vi "Create Data Row.vi"(0 "TestRunning?":bool, 1 "Steps":i32, 2 "StepIndex":i32, 3 "SkipStep":bool, 5 "DataCluster":T2, 7 "table.Data":string[][](array[string]), 9 "CommandCluster":T1, 11 "Controller?":bool, 12 "Serial Number":string) -> (4 "DataRow":string[](array[string]), 15 "LastDataTime":i64)   [LabVIEW 2013]
uses:
  TypeDef/DataCluster.ctl
  TypeDef/Command Cluster.ctl
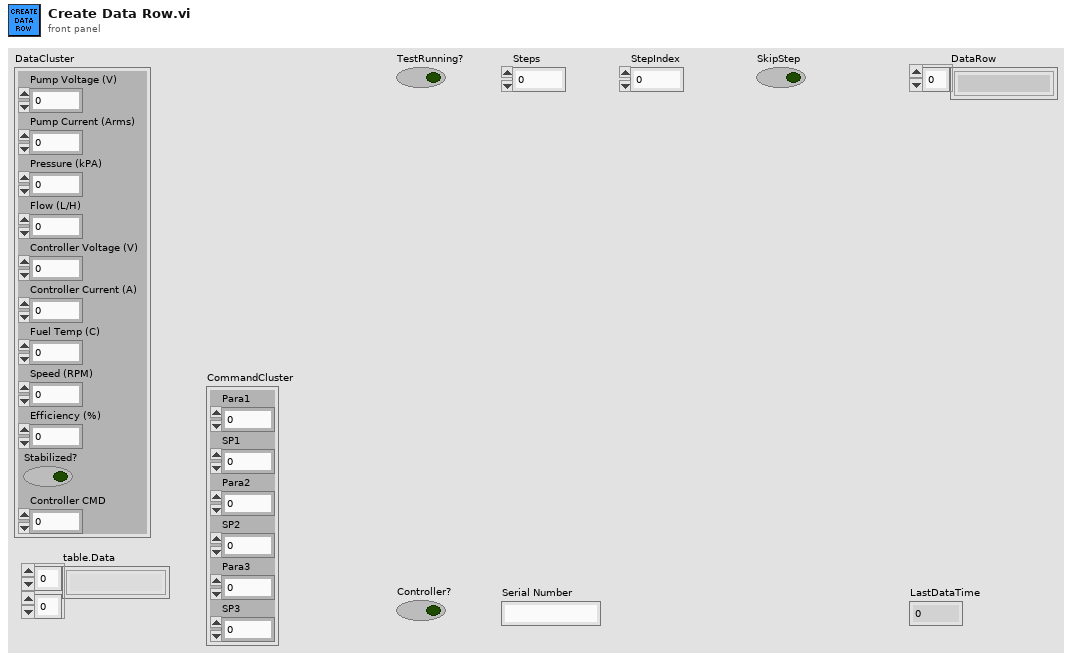
[diagram p1: front panel]
types:
  T1 = typedef "Command Cluster.ctl" = cluster{"Para1":i32, "SP1":dbl, "Para2":i32, "SP2":dbl, "Para3":i32, "SP3":dbl}
  T2 = typedef "DataCluster.ctl" = cluster{"Pump Voltage (V)":dbl, "Pump Current (Arms)":dbl, "Pressure (kPA)":dbl, "Flow (L/H)":dbl, "Controller Voltage (V)":dbl, "Controller Current (A)":dbl, "Fuel Temp (C)":dbl, "Speed (RPM)":dbl, "Efficiency (%)":dbl, "Stabilized?":bool, "Controller CMD":dbl}
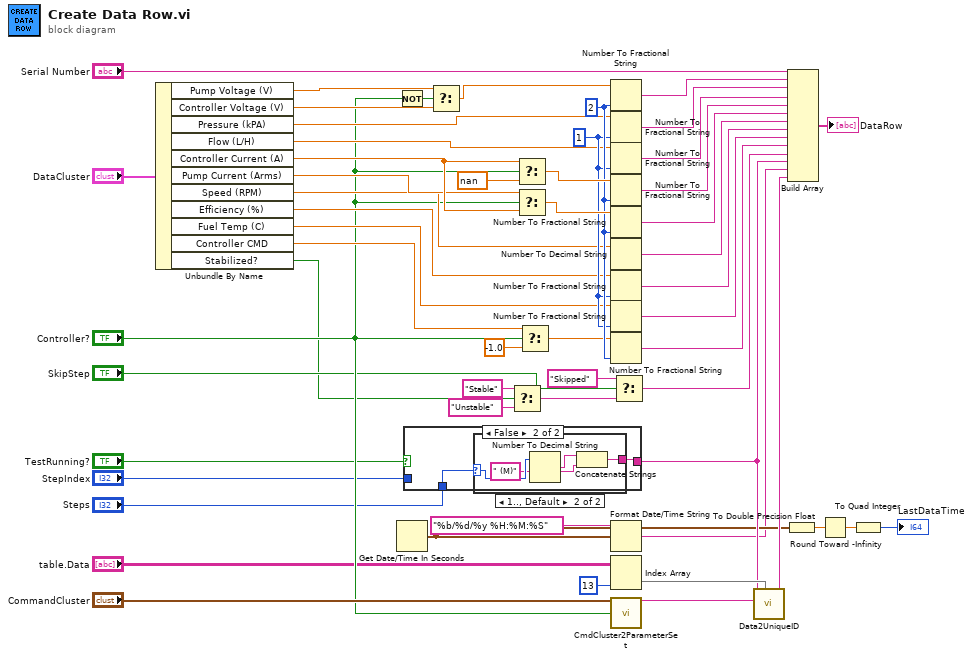
[diagram p0: block diagram]
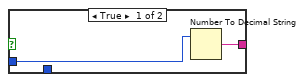
[diagram p2: hidden frame]
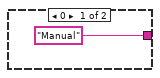
[diagram p3: hidden frame]
diagram:
  w35 = i16 1 ("precision (6)")
  w37 = i16 2 ("precision (6)")
  n1 = Unbundle By Name("DataCluster") -> ("Pump Voltage (V)"=w20:dbl, "Controller Voltage (V)"=w19:dbl, "Pressure (kPA)"=w18:dbl, "Flow (L/H)"=w17:dbl, "Controller Current (A)"=w16:dbl, "Pump Current (Arms)"=w15:dbl, "Speed (RPM)"=w14:dbl, "Efficiency (%)"=w13:dbl, "Fuel Temp (C)"=w12:dbl, "Controller CMD"=w11:dbl, "Stabilized?"=w1:bool)
  n2 = Not(x="Controller?") -> (.not. x?=w54:bool)
  n3 = Get Date/Time In Seconds() -> (seconds since 1Jan1904=w46:timestamp)
  n4 = case shown="False" "TestRunning?" {
    tunnel: "StepIndex" -> [w56 _]
    tunnel: [w57 w59] -> w52
    tunnel: "Steps" -> [_ w58]
    frame True {
      n5 = Number To Decimal String(number=w56) -> (decimal integer string=w57:string)  [unwired: 1 in]
    }
    frame False {
      n6 = case shown="1.., Default" w58 {
        selector: w58 -> [_ w62]
        tunnel: ["Manual" w63] -> w59
        frame 0 {
        }
        frame 1.., Default {
          n7 = Number To Decimal String(number=w62) -> (decimal integer string=w64:string)  [unwired: 1 in]
          n8 = Concatenate Strings(w64, " (M)") -> (w63:string)
        }
      }
    }
  }
  n9 = Select(t=w20, s=w54, f=w19) -> (s? t:f=w29:dbl)
  n10 = Select(t="Stable", s=w1, f="Unstable") -> (s? t:f=w31:string)
  n11 = Select(t=w16, s="Controller?", f=nan) -> (s? t:f=w48:dbl)
  n12 = Select(t=w15, s="Controller?", f=w16) -> (s? t:f=w49:dbl)
  n13 = Select(t=w11, s="Controller?", f=-1.0) -> (s? t:f=w28:dbl)
  n14 = Number To Fractional String(number=w29, precision (6)=w37) -> (F-format string=w23:string)  [unwired: 2 in]
  n15 = Number To Fractional String(number=w18, precision (6)=w35) -> (F-format string=w33:string)  [unwired: 2 in]
  n16 = Number To Fractional String(number=w17, precision (6)=w35) -> (F-format string=w34:string)  [unwired: 2 in]
  n17 = Number To Fractional String(number=w48, precision (6)=w37) -> (F-format string=w24:string)  [unwired: 2 in]
  n18 = Number To Fractional String(number=w49, precision (6)=w37) -> (F-format string=w38:string)  [unwired: 2 in]
  n19 = Number To Decimal String(number=w14) -> (decimal integer string=w36:string)  [unwired: 1 in]
  n20 = Number To Fractional String(number=w13, precision (6)=w35) -> (F-format string=w39:string)  [unwired: 2 in]
  n21 = Number To Fractional String(number=w12, precision (6)=w35) -> (F-format string=w40:string)  [unwired: 2 in]
  n22 = Number To Fractional String(number=w28, precision (6)=w37) -> (F-format string=w41:string)  [unwired: 2 in]
  n23 = Format Date/Time String(time format string (%c)="%b/%d/%y %H:%M:%S", seconds (now)=w46) -> (date/time string=w42:string)  [unwired: 1 in]
  n24 = Index Array(array="table.Data", index (col)=13 ("disabled index (col)")) -> (element=w55:string[])  [unwired: 1 in]
  n25 = call "CmdCluster2ParameterSet.vi"("CMDCluster"="CommandCluster", "Controller?"="Controller?") -> ("ParameterSet"=w51:string)  [unwired: 13 in]
  n26 = Select(t="Skipped", s="SkipStep", f=w31) -> (s? t:f=w32:string)
  n27 = call "Data2UniqueID.vi"("[UniqueID]s"=w55, "ParameterSet"=w51, "Step"=w52) -> ("UniqueID"=w53:string)  [unwired: 8 in]
  n28 = To Double Precision Float(number=w46) -> (double precision float=w45:dbl)
  n29 = Build Array("Serial Number", w23, w33, w34, w24, w38, w36, w39, w40, w41, w32, w52, w42, w53) -> (→"DataRow":string[])
  n30 = Round Toward -Infinity(1:w45) -> (0:w44:dbl)
  n31 = To Quad Integer(1:w44) -> (0:→"LastDataTime":i64)
